vi "Close.vi"(8 "error in":errorcluster, 11 "Modbus instance in":refnum<class "Modbus API.lvclass">) -> (0 "error out":errorcluster)   [LabVIEW 2014, in "T3110 & T2114.lvlib"]
uses:
  T3110 & T2114.lvlib
  <vilib>/NI/Modbus Library/API/Modbus API.lvclass
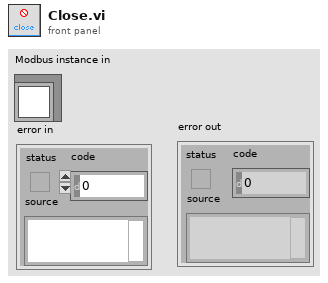
[diagram p1: front panel]
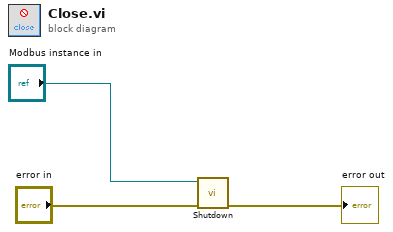
[diagram p0: block diagram]
diagram:
  n1 = call-dynamic "Shutdown.vi"("error in"="error in", "Modbus instance in"="Modbus instance in") -> ("error out"=→"error out":errorcluster)  [unwired: 9 in]
